vi "test Parse Push.vi"() -> (0 "error out":errorcluster, 2 "pass?":bool)   [LabVIEW 2019, in "RESP3 Tests.lvlib"]
uses:
  RESP3 Tests.lvlib
  RESP3/RESP3 Parser/RESP3 Parser.lvclass
  RESP3/types/RESP3 Type.ctl
  RESP3/types/RESP3 data type attribute.vi
  RESP3/RESP3.lvlib
  RESP3/high-level/RESP3 Get Array.vi
panel:
  out "RESP3 Value":variant
  out "finished?":bool
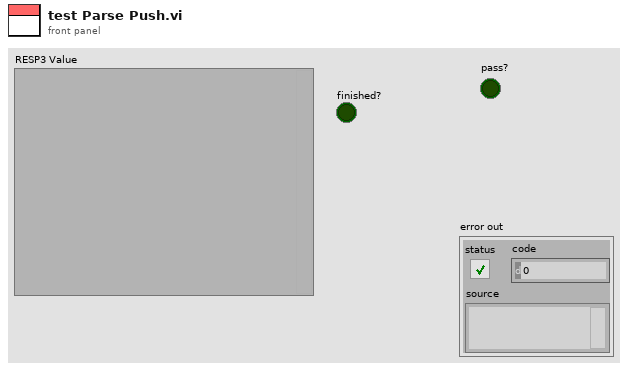
[diagram p1: front panel]
types:
  T1 = typedef "RESP3.lvlib/RESP3 Type.ctl" = enum8{"<0x00>", "<0x01>", "<0x02>", "<0x03>", "<0x04>", "<0x05>", "<0x06>", "<0x07>", "<0x08>", "<0x09>", "<0x0A>", "<0x0B>", "<0x0C>", "<0x0D>", "<0x0E>", "<0x0F>", "<0x10>", "<0x11>", "<0x12>", "<0x13>", "<0x14>", "<0x15>", "<0x16>", "<0x17>", "<0x18>", "<0x19>", "<0x1A>", "<0x1B>", "<0x1C>", "<0x1D>", "<0x1E>", "<0x1F>", "\" \"", "BLOB ERROR", "\"\"\"", "BOOLEAN", "BLOB", "MAP", "\"&\"", "\"'\"", "BIG NUMBER", "\")\"", "ARRAY", "STRING", "DOUBLE", "ERROR", "END", "\"/\"", "\"0\"", "\"1\"", "\"2\"", "\"3\"", "\"4\"", "\"5\"", "\"6\"", "\"7\"", "\"8\"", "\"9\"", "INTEGER", "STREAM", "\"<\"", "VERBATIM STRING", "PUSH", "\"?\"", "\"@\"", "\"A\"", "\"B\"", "\"C\"", "\"D\"", "\"E\"", "\"F\"", "\"G\"", "\"H\"", "\"I\"", "\"J\"", "\"K\"", "\"L\"", "\"M\"", "\"N\"", "\"O\"", "\"P\"", "\"Q\"", "\"R\"", "\"S\"", "\"T\"", "\"U\"", "\"V\"", "\"W\"", "\"X\"", "\"Y\"", "\"Z\"", "\"[\"", "\"\\\"", "\"]\"", "\"^\"", "NULL", "\"`\"", "\"a\"", "\"b\"", "\"c\"", "\"d\"", "\"e\"", "\"f\"", "\"g\"", "\"h\"", "\"i\"", "\"j\"", "\"k\"", "\"l\"", "\"m\"", "\"n\"", "\"o\"", "\"p\"", "\"q\"", "\"r\"", "\"s\"", "\"t\"", "\"u\"", "\"v\"", "\"w\"", "\"x\"", "\"y\"", "\"z\"", "\"{\"", "ATTRIBUTES", "\"}\"", "SET", "<0x7F>", "<0x80>", "<0x81>", "<0x82>", "<0x83>", "<0x84>", "<0x85>", "<0x86>", "<0x87>", "<0x88>", "<0x89>", "<0x8A>", "<0x8B>", "<0x8C>", "<0x8D>", "<0x8E>", "<0x8F>", "<0x90>", "<0x91>", "<0x92>", "<0x93>", "<0x94>", "<0x95>", "<0x96>", "<0x97>", "<0x98>", "<0x99>", "<0x9A>", "<0x9B>", "<0x9C>", "<0x9D>", "<0x9E>", "<0x9F>", "<0xA0>", "<0xA1>", "<0xA2>", "<0xA3>", "<0xA4>", "<0xA5>", "<0xA6>", "<0xA7>", "<0xA8>", "<0xA9>", "<0xAA>", "<0xAB>", "<0xAC>", "<0xAD>", "<0xAE>", "<0xAF>", "<0xB0>", "<0xB1>", "<0xB2>", "<0xB3>", "<0xB4>", "<0xB5>", "<0xB6>", "<0xB7>", "<0xB8>", "<0xB9>", "<0xBA>", "<0xBB>", "<0xBC>", "<0xBD>", "<0xBE>", "<0xBF>", "<0xC0>", "<0xC1>", "<0xC2>", "<0xC3>", "<0xC4>", "<0xC5>", "<0xC6>", "<0xC7>", "<0xC8>", "<0xC9>", "<0xCA>", "<0xCB>", "<0xCC>", "<0xCD>", "<0xCE>", "<0xCF>", "<0xD0>", "<0xD1>", "<0xD2>", "<0xD3>", "<0xD4>", "<0xD5>", "<0xD6>", "<0xD7>", "<0xD8>", "<0xD9>", "<0xDA>", "<0xDB>", "<0xDC>", "<0xDD>", "<0xDE>", "<0xDF>", "<0xE0>", "<0xE1>", "<0xE2>", "<0xE3>", "<0xE4>", "<0xE5>", "<0xE6>", "<0xE7>", "<0xE8>", "<0xE9>", "<0xEA>", "<0xEB>", "<0xEC>", "<0xED>", "<0xEE>", "<0xEF>", "<0xF0>", "<0xF1>", "<0xF2>", "<0xF3>", "<0xF4>", "<0xF5>", "<0xF6>", "<0xF7>", "<0xF8>", "<0xF9>", "<0xFA>", "<0xFB>", "<0xFC>", "<0xFD>", "<0xFE>"}
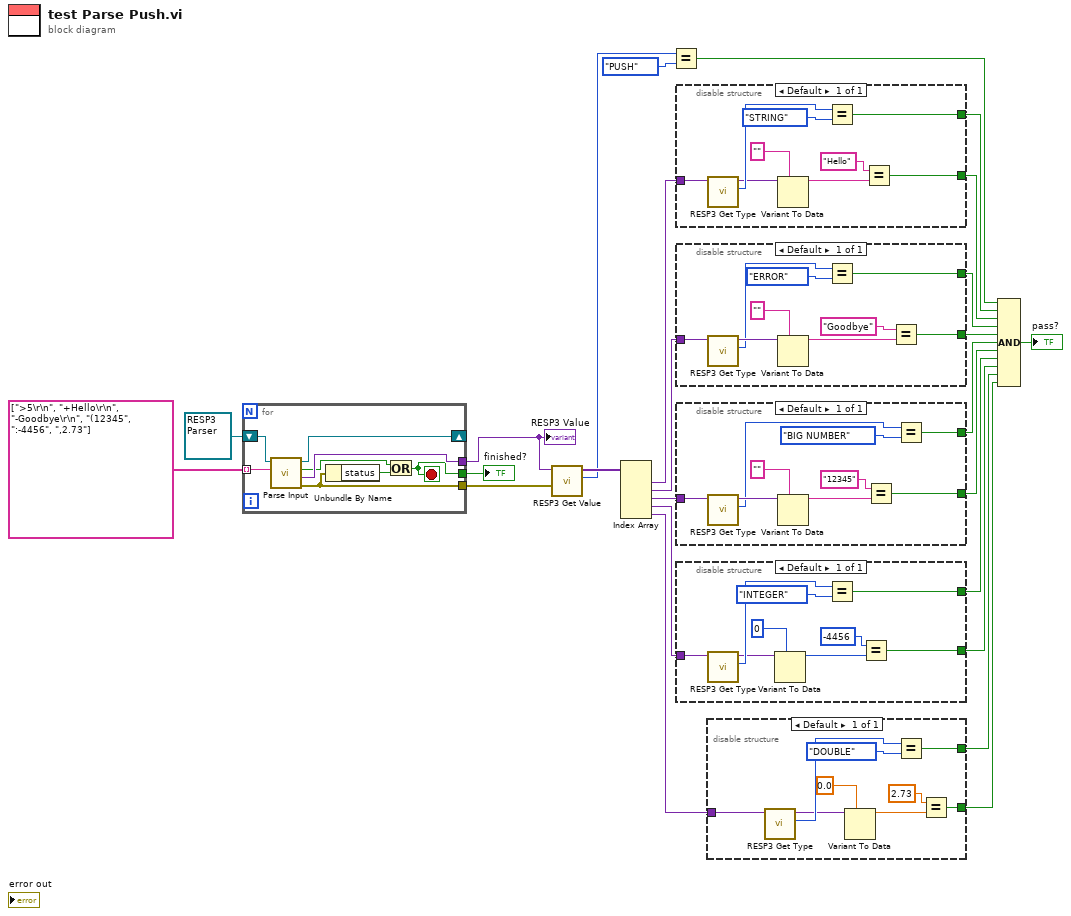
[diagram p0: block diagram]
diagram:
  n1 = for {
    shift-right: [w32] -> _
    shift-left: refnum<class "RESP3 Parser.lvclass"> refnum ("RESP3.lvlib:RESP3 Parser.lvclass") -> [w33]
    tunnel: string[] [">5\r\n", "+Hello\r\n", "-Goodbye\r\n", "(12345", ":-4456", ",2.73"] -> [w31] mode=indexing
    tunnel: [w30] -> w4
    tunnel: [w28] -> w23
    tunnel: [w26] -> w3
    stop <- w28 stop-if-true
    n2 = call-dynamic "Parse Input.vi"("input line"=w31, "RESP3 Parser in"=w33) -> ("error out"=w26:errorcluster, "RESP3 Value"=w30:variant, "finished?"=w29:bool, "RESP3 Parser out"=w32:refnum<class "RESP3 Parser.lvclass">)  [unwired: 5 in, 1 out]
    n3 = Unbundle By Name(w26) -> ("status"=w27:bool)
    n4 = Or(x=w29, y=w27) -> (x .or. y?=w28:bool)
  }
  "finished?" <- w23
  "RESP3 Value" <- w4
  n5 = call-poly "RESP3 Get Value.vi"("error in (no error)"=w3, "RESP3 Value in"=w4) -> ("actual RESP3 type"=w1:T1, "RESP3 Values out"=w2:variant[])  [unwired: 6 in, 2 out]
  n6 = Index Array(array=w2) -> (element #1=w20:variant, element #2=w17:variant, element #3=w13:variant, element #4=w9:variant, element #5=w10:variant)  [unwired: 5 in]
  n7 = Equal?(x=w1, y=RESP3_Type."PUSH") -> (x = y?=w21:bool)
  n8 = disable-structure shown="Default" {
    disable-tunnel: w20 -> [w42]
    disable-tunnel: [w39] -> w19
    disable-tunnel: [w34] -> w18
    frame Enabled {
      n9 = call "RESP3 Get Type.vi"("RESP3 Value in"=w42) -> ("RESP3 Type"=w40:T1, "RESP3 Value out"=w38:variant)  [unwired: 7 in, 2 out]
      n10 = Variant To Data(type="", Variant=w38) -> (data=w36:string)  [unwired: 1 in, 1 out]
      n11 = Equal?(x=w40, y=RESP3_Type."STRING") -> (x = y?=w39:bool)
      n12 = Equal?(x="Hello", y=w36) -> (x = y?=w34:bool)
    }
  }
  n13 = disable-structure shown="Default" {
    disable-tunnel: w17 -> [w45]
    disable-tunnel: [w44] -> w16
    disable-tunnel: [w43] -> w15
    frame Enabled {
      n14 = call "RESP3 Get Type.vi"("RESP3 Value in"=w45) -> ("RESP3 Type"=w48:T1, "RESP3 Value out"=w49:variant)  [unwired: 7 in, 2 out]
      n15 = Variant To Data(type="", Variant=w49) -> (data=w50:string)  [unwired: 1 in, 1 out]
      n16 = Equal?(x=w48, y=RESP3_Type."ERROR") -> (x = y?=w44:bool)
      n17 = Equal?(x="Goodbye", y=w50) -> (x = y?=w43:bool)
    }
  }
  n18 = disable-structure shown="Default" {
    disable-tunnel: w13 -> [w54]
    disable-tunnel: [w53] -> w12
    disable-tunnel: [w52] -> w11
    frame Enabled {
      n19 = call "RESP3 Get Type.vi"("RESP3 Value in"=w54) -> ("RESP3 Type"=w57:T1, "RESP3 Value out"=w58:variant)  [unwired: 7 in, 2 out]
      n20 = Variant To Data(type="", Variant=w58) -> (data=w59:string)  [unwired: 1 in, 1 out]
      n21 = Equal?(x="12345", y=w59) -> (x = y?=w52:bool)
      n22 = Equal?(x=w57, y=RESP3_Type."BIG NUMBER") -> (x = y?=w53:bool)
    }
  }
  n23 = disable-structure shown="Default" {
    disable-tunnel: [w67] -> w8
    disable-tunnel: [w61] -> w7
    disable-tunnel: w9 -> [w65]
    frame Enabled {
      n24 = call "RESP3 Get Type.vi"("RESP3 Value in"=w65) -> ("RESP3 Type"=w68:T1, "RESP3 Value out"=w66:variant)  [unwired: 7 in, 2 out]
      n25 = Variant To Data(type=i64 0, Variant=w66) -> (data=w63:i64)  [unwired: 1 in, 1 out]
      n26 = Equal?(x=w68, y=RESP3_Type."INTEGER") -> (x = y?=w67:bool)
      n27 = Equal?(x=i64 -4456, y=w63) -> (x = y?=w61:bool)
    }
  }
  n28 = disable-structure shown="Default" {
    disable-tunnel: [w76] -> w6
    disable-tunnel: [w70] -> w5
    disable-tunnel: w10 -> [w74]
    frame Enabled {
      n29 = call "RESP3 Get Type.vi"("RESP3 Value in"=w74) -> ("RESP3 Type"=w77:T1, "RESP3 Value out"=w75:variant)  [unwired: 7 in, 2 out]
      n30 = Variant To Data(type=0.0, Variant=w75) -> (data=w72:dbl)  [unwired: 1 in, 1 out]
      n31 = Equal?(x=w77, y=RESP3_Type."DOUBLE") -> (x = y?=w76:bool)
      n32 = Equal?(x=2.73, y=w72) -> (x = y?=w70:bool)
    }
  }
  n33 = Compound Arithmetic op=AND(w21, w19, w18, w16, w15, w12, w11, w8, w7, w6, w5) -> (→"pass?":bool)
